vi "Is Error.vi"(8 "Error In":errorcluster) -> (0 "Error Out":errorcluster)   [LabVIEW 2017, in "Tests.lvlib" / "Reader.lvlib"]
uses:
  Reader.lvlib
  src/LabPack/Public/Reader/Reader.lvclass/Reader.ctl
  <vilib>/addons/_JKI Toolkits/Caraya/classes/Test/Test.lvclass
  src/LabPack/Public/Reader/Reader.lvclass
  <vilib>/addons/_JKI Toolkits/Caraya/classes/Assert/Assert.lvclass
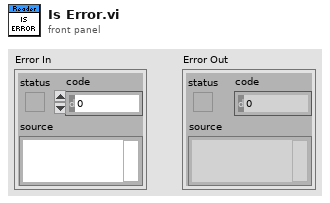
[diagram p1: front panel]
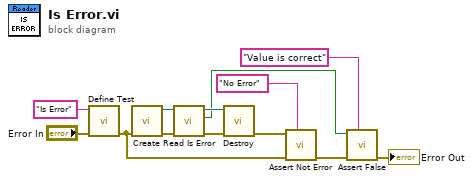
[diagram p0: block diagram]
diagram:
  n1 = call <vilib>:"Define Test.vi"("error in (no error)"="Error In", "Label (VI Title)"="Is Error") -> ("error out"=w2:errorcluster)  [unwired: 9 in]
  n2 = call "Create.vi"("Error In"=w2) -> ("Error Out"=w10:errorcluster, "Reader"=w11:refnum<class "Reader.lvclass">)  [unwired: 9 in]
  n3 = call "Read Is Error.vi"("Error In"=w10, "Reader In"=w11) -> ("Error Out"=w8:errorcluster, "Error"=w5:bool, "Reader Out"=w9:refnum<class "Reader.lvclass">)  [unwired: 7 in]
  n4 = call "Destroy.vi"("Error In"=w8, "Reader"=w9) -> ("Error Out"=w7:errorcluster)  [unwired: 9 in]
  n5 = call <vilib>:"Assert Not Error.vi"("Label"="No Error", "error in (no error)"=w2, "Not Error?"=w7) -> ("error out"=w3:errorcluster)  [unwired: 8 in]
  n6 = call <vilib>:"Assert False.vi"("Label"="Value is correct", "error in (no error)"=w3, "False?"=w5) -> ("error out"=→"Error Out":errorcluster)  [unwired: 8 in]
